vi "Generate ID.vi"() -> (3 "ID":string)   [LabVIEW 2013, in "ControlPacket.lvclass"]
uses:
  ControlPacket.lvclass
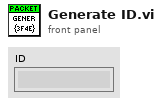
[diagram p1: front panel]
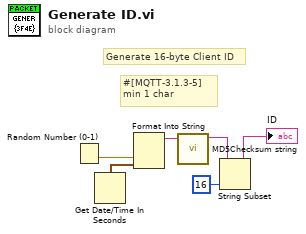
[diagram p0: block diagram]
diagram:
  # "#[MQTT-3.1.3-5]\nmin 1 char"
  # "Generate 16-byte Client ID"
  n1 = Random Number (0-1)() -> (number: 0 to 1=w2:dbl)
  n2 = Get Date/Time In Seconds() -> (seconds since 1Jan1904=w3:timestamp)
  n3 = Format Into String(w2, w3) -> (resulting string=w1:string)  [unwired: 3 in, 1 out]
  n4 = call <vilib>:"MD5Checksum string.vi"("Message String"=w1) -> ("MD5 message-digest"=w4:string)  [unwired: 10 in]
  n5 = String Subset(string=w4, length (rest)=16 ("length (rest)")) -> (substring=→"ID":string)  [unwired: 1 in]
